vi "Do I Upshift.vi"(8 "Cluster":T1) -> (5 "Enum":T3)   [LabVIEW 2013]
uses:
  Drive Train States.ctl
  Drive Train Metrics.ctl
  CmdFlag.ctl
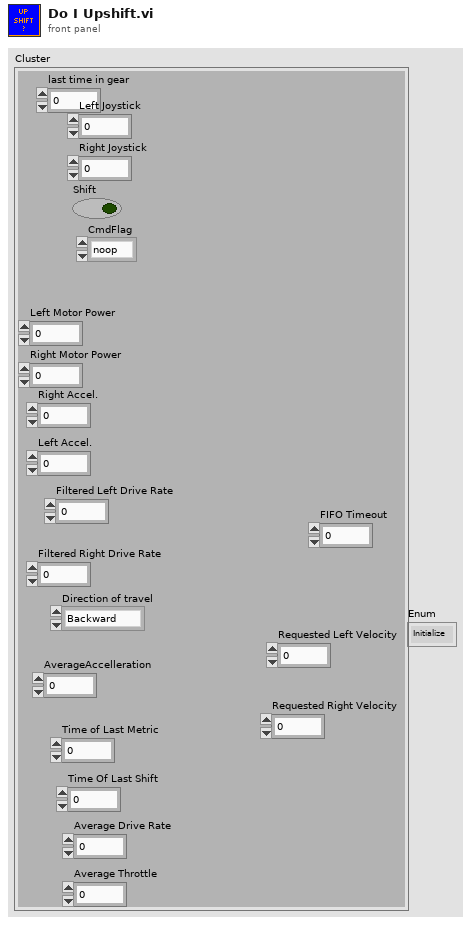
[diagram p1: front panel]
types:
  T1 = typedef "Drive Train Metrics.ctl" = cluster{"last time in gear":u32, "Shift":bool, "Right Joystick":dbl, "Left Joystick":dbl, "CmdFlag":T2, "Right Motor Power":dbl, "Left Motor Power":dbl, "Right Accel.":dbl, "Left Accel.":dbl, "Filtered Left Drive Rate":dbl, "Filtered Right Drive Rate":dbl, "Direction of travel":enum16{"Backward", "Forward", "Spin"}, "AverageAccelleration":dbl, "Time of Last Metric":u32, "Time Of Last Shift":dbl, "Average Drive Rate":dbl, "Average Throttle":dbl, "FIFO Timeout":i32, "Requested Left Velocity":dbl, "Requested Right Velocity":dbl}
  T2 = typedef "CmdFlag.ctl" = enum16{"noop", "suspend", "resume"}
  T3 = typedef "Drive Train States.ctl" = enum16{"Initialize", "Low_gear", "Upshift", "Wait For Upshift", "Upshift Complete", "High_gear", "Downshift", "Wait For Downshift", "Downshift Complete", "Suspend", "Resume"}
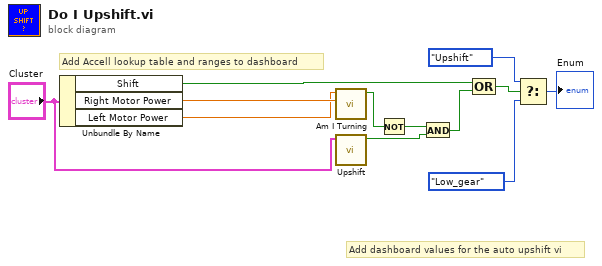
[diagram p0: block diagram]
diagram:
  # "Add dashboard values for the auto upshift vi"
  # "Add Accell lookup table and ranges to dashboard"
  n1 = Unbundle By Name("Cluster") -> ("Shift"=w9:bool, "Right Motor Power"=w7:dbl, "Left Motor Power"=w6:dbl)
  n2 = call "Am I Turning.vi"("Right Joystick"=w7, "Left Joystick"=w6) -> ("Turn?"=w3:bool)  [unwired: 9 in]
  n3 = call "Upshift.vi"("Cluster"="Cluster") -> ("Upshift?"=w4:bool)  [unwired: 10 in]
  n4 = Not(x=w3) -> (.not. x?=w2:bool)
  n5 = And(x=w2, y=w4) -> (x .and. y?=w5:bool)
  n6 = Compound Arithmetic op=OR(w9, w5) -> (w8:bool)
  n7 = Select(t=Drive_Train_States."Upshift", s=w8, f=Drive_Train_States."Low_gear") -> (s? t:f=→"Enum":T3)
